vi "Host sender&receiver.vi"() -> ()   [LabVIEW 2017]
panel:
  out "Rx unflattened":T1
  out "Received String from myRIO":string
  in  "stop":bool
  out "Sent Number to myRIO":string
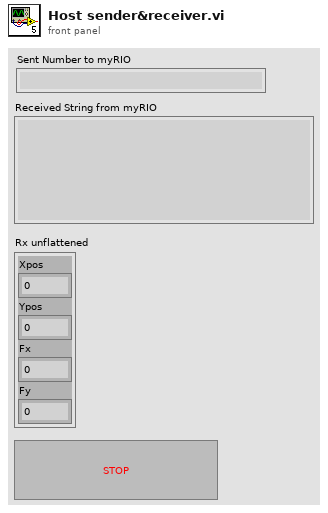
[diagram p1: front panel]
types:
  T1 = cluster{"Xpos":dbl, "Ypos":dbl, "Fx":dbl, "Fy":dbl}
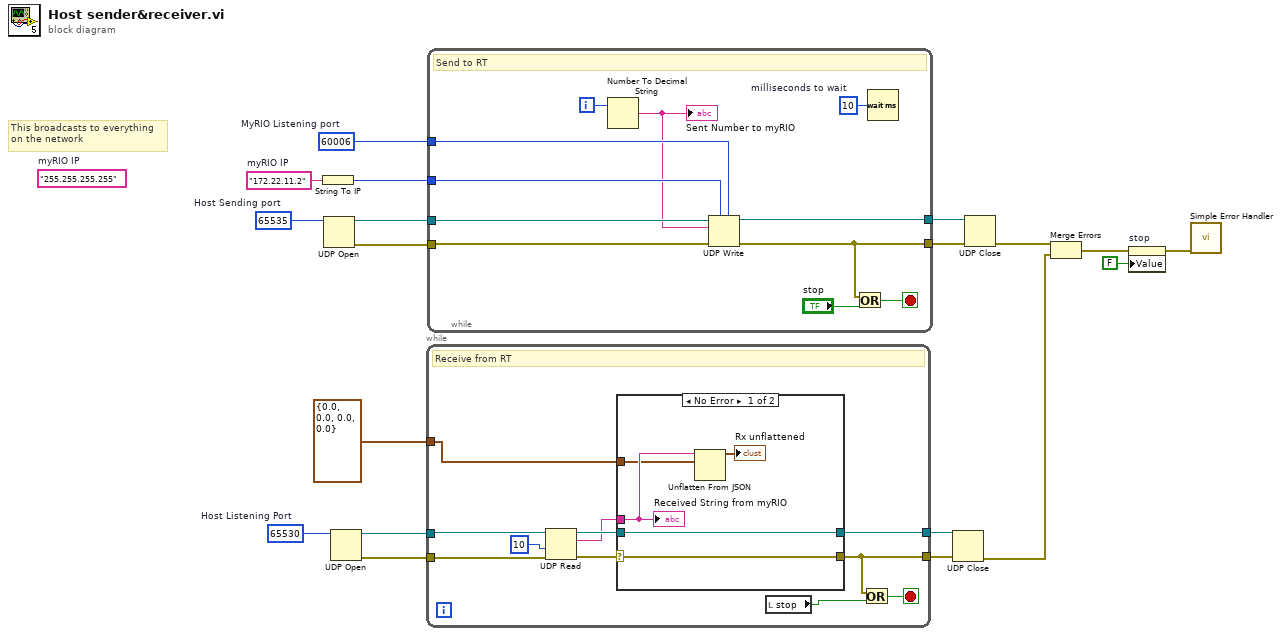
[diagram p0: block diagram]
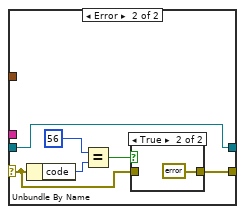
[diagram p2: hidden frame]
diagram:
  w2 = "172.22.11.2"  # myRIO IP
  w10 = u16 65530  # Host Listening Port
  w15 = u16 60006  # MyRIO Listening port
  (unwired) "255.255.255.255"  # myRIO IP
  w19 = u16 65535  # Host Sending port
  # "This broadcasts to everything\non the network"
  n1 = String To IP(1:w2) -> (0:w16:u32)
  n2 = UDP Open(11:w19) -> (port=w17:refnum<k16>, 0:w18:errorcluster)  [unwired: 4 in, 1 out]
  n3 = UDP Open(11:w10) -> (port=w12:refnum<k16>, 0:w11:errorcluster)  [unwired: 4 in, 1 out]
  n4 = while {
    tunnel: w12 -> [w30]
    tunnel: w11 -> [w29]
    tunnel: [w22] -> w9
    tunnel: [w24] -> w8
    tunnel: T1 {"Xpos"=0.0, "Ypos"=0.0, "Fx"=0.0, "Fy"=0.0} -> [w20]
    stop <- w23 stop-if-true
    # "Receive from RT"
    n5 = UDP Read(connection ID=w30, timeout ms (25000)=10, 8:w29) -> (data out=w25:string, error out=w27:errorcluster, 3:w26:refnum<k16>)  [unwired: 1 in, 2 out]
    n6 = case shown="No Error" w27 {
      selector: w27 -> [w35 w37]
      tunnel: w26 -> [w34 w36]
      tunnel: w25 -> [w33 _]
      tunnel: [w35 w38] -> w22
      tunnel: [w34 w36] -> w24
      tunnel: w20 -> [w32 _]
      frame No Error {
        n7 = Unflatten From JSON(JSON string=w33, type and defaults=w32) -> (value=→"Rx unflattened":T1)  [unwired: 5 in, 1 out]
        "Received String from myRIO" <- w33
      }
      frame Error {
        n8 = Unbundle By Name(w37) -> ("code"=w41:i32)
        n9 = Equal?(x=56, y=w41) -> (x = y?=w39:bool)
        n10 = case shown="True" w39 {
          tunnel: [w42 errorcluster {"status"=FALSE, "code"=0, "source"=""} ("error constant")] -> w38
          tunnel: w37 -> [w42 _]
          frame False {
          }
          frame True {
          }
        }
      }
    }
    n11 = local read "stop"() -> (w21:bool)
    n12 = Or(x=w22, y=w21) -> (x .or. y?=w23:bool)
  }
  n13 = while {
    tunnel: w18 -> [w52]
    tunnel: w17 -> [w53]
    tunnel: w16 -> [w51]
    tunnel: w15 -> [w50]
    tunnel: [w47] -> w14
    tunnel: [w45] -> w13
    i -> [w49]
    stop <- w46 stop-if-true
    w54 = u32 10  # milliseconds to wait
    # "Send to RT"
    n14 = Number To Decimal String(number=w49) -> (decimal integer string=w48:string)  [unwired: 1 in]
    "Sent Number to myRIO" <- w48
    n15 = UDP Write(address=w51, port or service name=w50, connection ID=w53, data in=w48, 8:w52) -> (error out=w45:errorcluster, 3:w47:refnum<k16>)  [unwired: 1 in]
    n16 = Or(x=w45, y="stop") -> (x .or. y?=w46:bool)
    n17 = Wait (ms)(milliseconds to wait=w54) -> ()  [unwired: 1 out]
  }
  n18 = UDP Close(connection ID=w8, 8:w9) -> (error out=w6:errorcluster)  [unwired: 1 out]
  n19 = UDP Close(connection ID=w14, 8:w13) -> (error out=w7:errorcluster)  [unwired: 1 out]
  n20 = Merge Errors(w7, w6) -> (w5:errorcluster)
  n21 = property on="stop" class="Bool (strict)"(error in=w5, "Value"=FALSE ("stop")) -> (error out=w4:errorcluster)  [unwired: 1 in, 1 out]
  n22 = call <vilib>:"Simple Error Handler.vi"("error in (no error)"=w4) -> ()  [unwired: 4 in, 5 out]
